vi "Cumulative Histogram.vi"() -> ()   [LabVIEW 2020]
doc: "VI che calcola l'istogramma dell'immagine"
panel:
  in  "Tab Control":enum32{"Immagini", "Istogrammi"}(tab)
  out "Gray level image INPUT":T1(plugin-control)
  in  "stop":bool
  in  "Path Image Load":path=path "C:/Users/Dell/Documents/Vision-System/Images/Iron.tif"
  in  "error in (no error)":errorcluster
  out "error out":errorcluster
  out "Input cumulative histogram":u32[](graph)
  out "Input Histohraph":T2(graph)
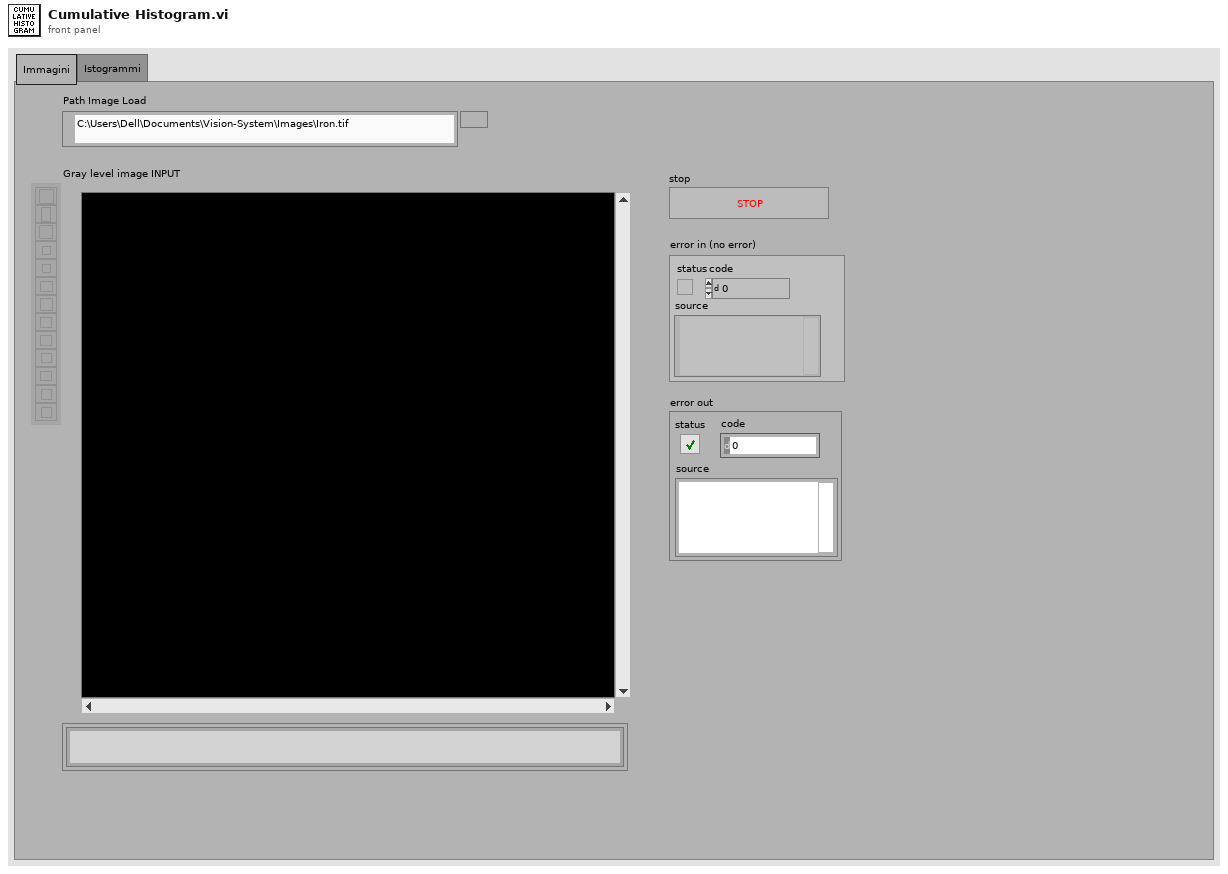
[diagram p1: front panel]
types:
  T1 = typedef "IMAQ Image.ctl" = refnum<image>
  T2 = cluster{"Starting Value":sgl, "Incremental Value":sgl, "Histogram":u32[]}
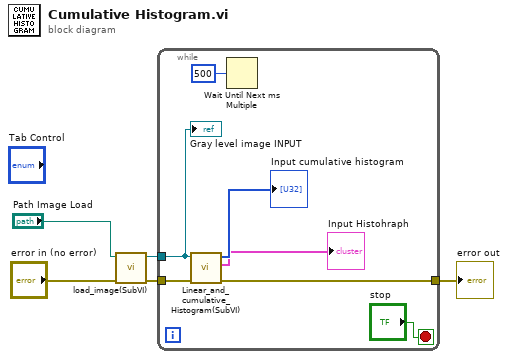
[diagram p0: block diagram]
diagram:
  n1 = call "load_image(SubVI).vi"("error in (no error)"="error in (no error)", "Image Path"="Path Image Load") -> ("error out"=w2:errorcluster, "Image GRAY"=w3:T1)  [unwired: 8 in]
  n2 = while {
    tunnel: w3 -> [w10]
    tunnel: w2 -> [w9]
    tunnel: [w6] -> w1
    stop <- "stop" stop-if-true
    n3 = call "Linear_and_cumulative_Histogram(SubVI).vi"("error in (no error)"=w9, "Image GRAY"=w10) -> ("error out"=w6:errorcluster, "Linear Histogram"=→"Input Histohraph":T2, "Cumulative Histogram"=→"Input cumulative histogram":u32[])  [unwired: 7 in]
    n4 = Wait Until Next ms Multiple(millisecond multiple=u32 500) -> ()  [unwired: 1 out]
    "Gray level image INPUT" <- w10
  }
  "error out" <- w1
